vi "camera_imaging_source_MAIN.vi"() -> ()   [LabVIEW 2024]
panel:
  out "Camera Ready":bool
  in  "Live":bool
  in  "Camera Properties":bool
  in  "Stop Camera":bool
  out "Image":T1(plugin-control)
  in  "ICImagingControl":refnum<k7>(container)
  in  "Configuration File Path":path
  in  "Grab Image":bool
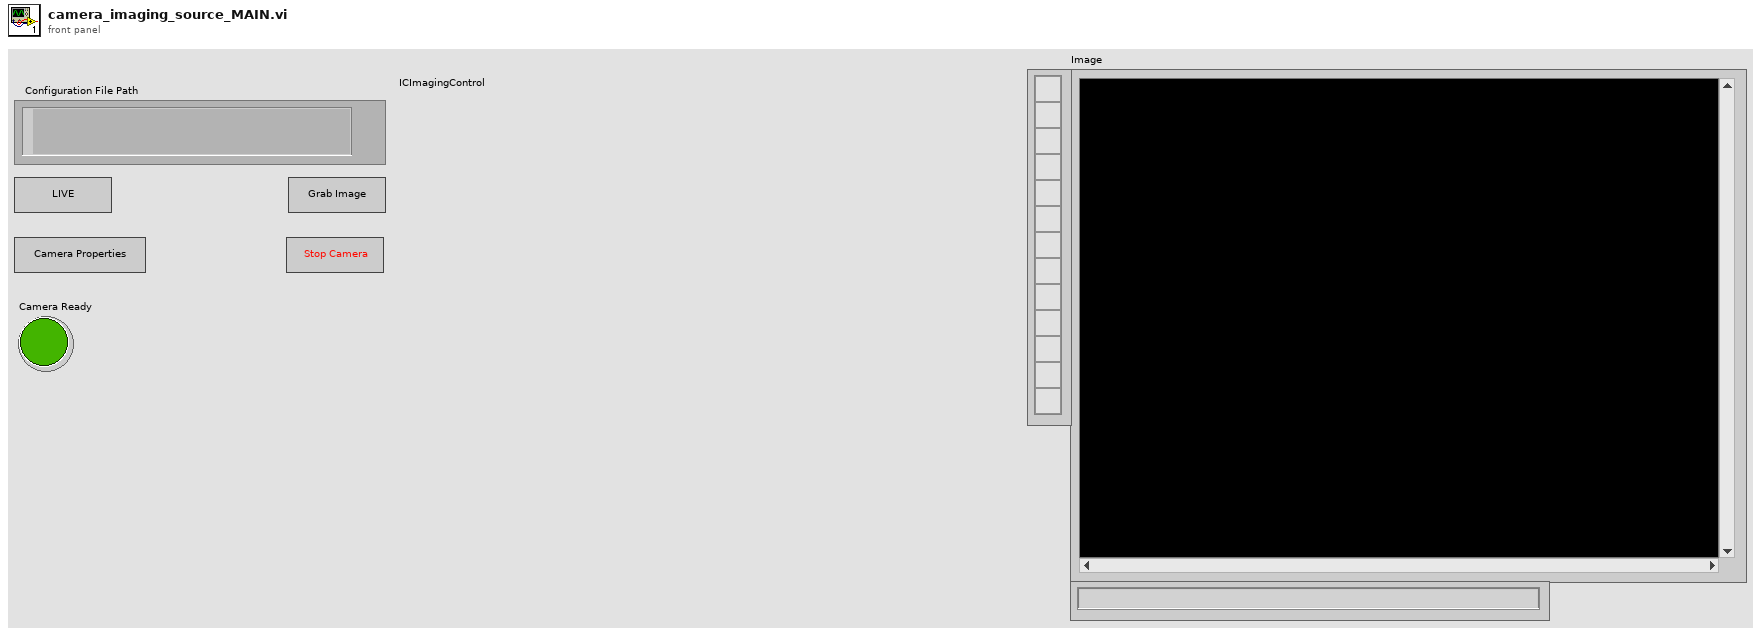
[diagram p1: front panel]
types:
  T1 = typedef "IMAQ Image.ctl" = refnum<image>
  T2 = enum16{"Init", "Idle", "Open Properties", "Grab Image", "Stop All", "Set Live"}
  T3 = enum16{"Init", "Idle", "Open Properties", "Grab Image", "Stop All"}
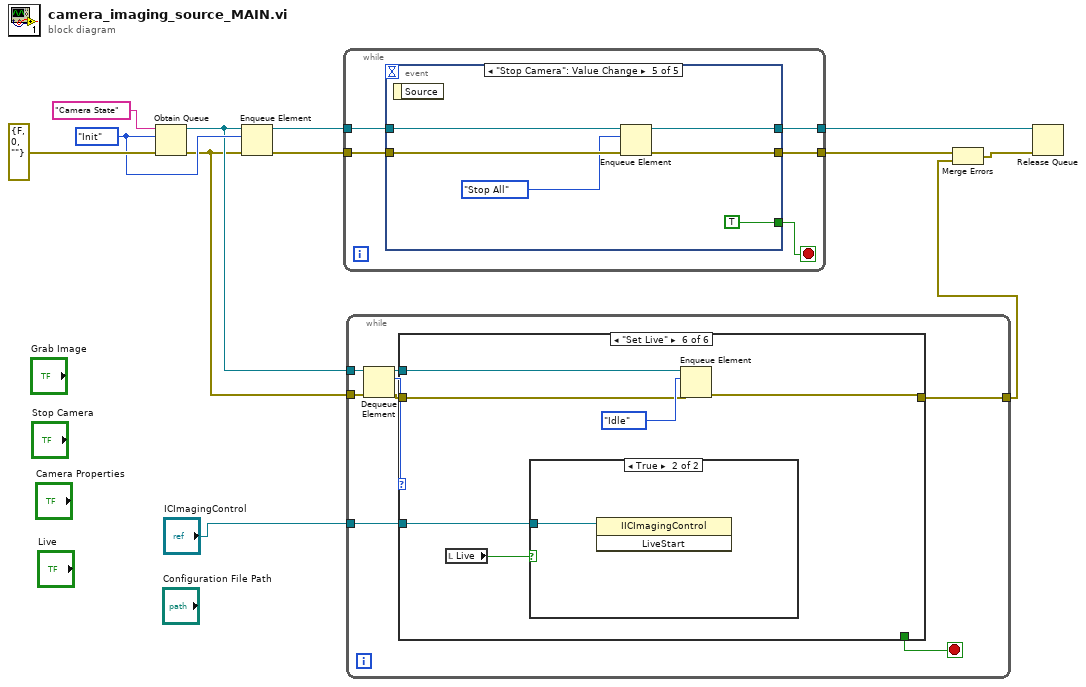
[diagram p0: block diagram]
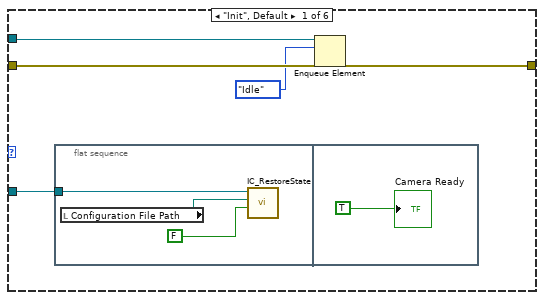
[diagram p2: hidden frame]
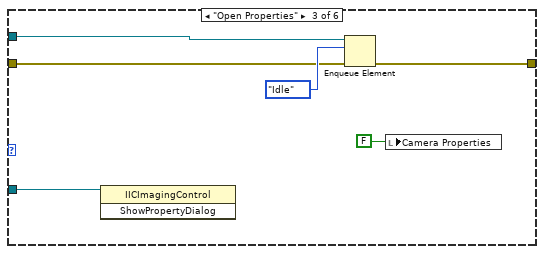
[diagram p4: hidden frame]
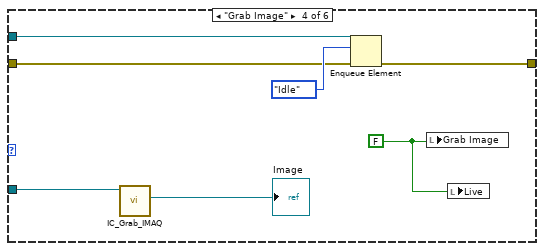
[diagram p5: hidden frame]
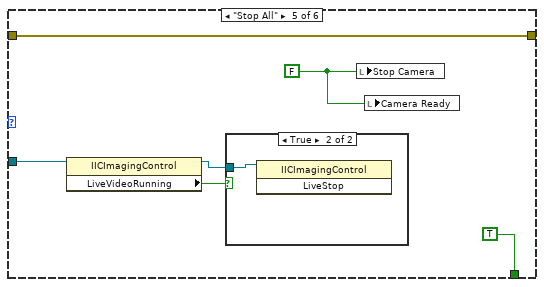
[diagram p6: hidden frame]
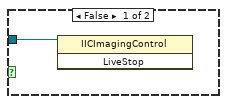
[diagram p8: hidden frame]
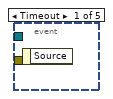
[diagram p9: hidden frame]
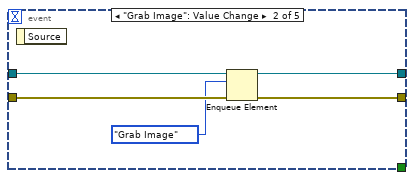
[diagram p10: hidden frame]
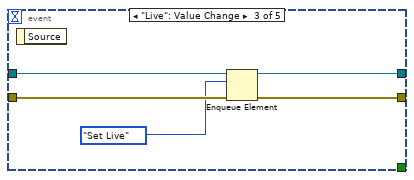
[diagram p11: hidden frame]
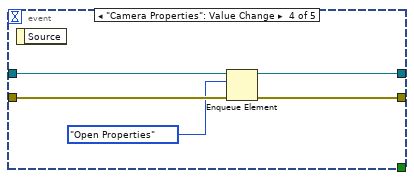
[diagram p12: hidden frame]
diagram:
  w10 = T2."Init"
  n1 = Obtain Queue(name (unnamed)="Camera State", element data type=w10, error in (no error)=errorcluster {"status"=FALSE, "code"=0, "source"=""}) -> (queue out=w9:refnum<queue>, error out=w8:errorcluster)  [unwired: 2 in, 1 out]
  n2 = Enqueue Element(queue=w9, element=w10, error in (no error)=w8) -> (queue out=w6:refnum<queue>, error out=w5:errorcluster)  [unwired: 1 in, 1 out]
  n3 = while {
    tunnel: w6 -> [w17]
    tunnel: w5 -> [w16]
    tunnel: [w15] -> w4
    tunnel: [w14] -> w2
    stop <- w13 stop-if-true
    n4 = event shown="[4] \"Stop Camera\": Value Change" {
      selector: _ -> [_ _ _ _ _]
      dyn-events: _ -> [_ _ _ _ _]
      timeout: _ -> [_ _ _ _ _]
      tunnel: w17 -> [_ w22 w27 w32 w37]
      tunnel: w16 -> [_ w21 w26 w31 w36]
      tunnel: [_ w19 w25 w29 w34] -> w15
      tunnel: [_ w18 w24 w28 w35] -> w14
      tunnel: [_ _ _ _ TRUE] -> w13
      event Timeout {
        n5 = event-data() -> ()  [unwired: 1 in, 1 out]
      }
      event "Grab Image": Value Change {
        n6 = event-data() -> ()  [unwired: 1 in, 1 out]
        n7 = Enqueue Element(queue=w22, element=T3."Grab Image", error in (no error)=w21) -> (queue out=w19:refnum<queue>, error out=w18:errorcluster)  [unwired: 1 in, 1 out]
      }
      event "Live": Value Change {
        n8 = event-data() -> ()  [unwired: 1 in, 1 out]
        n9 = Enqueue Element(queue=w27, element=T2."Set Live", error in (no error)=w26) -> (queue out=w25:refnum<queue>, error out=w24:errorcluster)  [unwired: 1 in, 1 out]
      }
      event "Camera Properties": Value Change {
        n10 = event-data() -> ()  [unwired: 1 in, 1 out]
        n11 = Enqueue Element(queue=w32, element=T3."Open Properties", error in (no error)=w31) -> (queue out=w29:refnum<queue>, error out=w28:errorcluster)  [unwired: 1 in, 1 out]
      }
      event "Stop Camera": Value Change {
        n12 = event-data() -> ()  [unwired: 1 in, 1 out]
        n13 = Enqueue Element(queue=w37, element=T3."Stop All", error in (no error)=w36) -> (queue out=w34:refnum<queue>, error out=w35:errorcluster)  [unwired: 1 in, 1 out]
      }
    }
  }
  n14 = while {
    tunnel: w9 -> [w46]
    tunnel: w8 -> [w45]
    tunnel: "ICImagingControl" -> [w43]
    tunnel: [w42] -> w3
    stop <- w40 stop-if-true
    n15 = Dequeue Element(queue=w46, error in (no error)=w45) -> (queue out=w39:refnum<queue>, element=w44:T2, error out=w41:errorcluster)  [unwired: 1 in, 1 out]
    n16 = case shown="\"Set Live\"" w44 {
      tunnel: w43 -> [w47 _ w62 w69 w74 w82]
      tunnel: [w50 w56 w58 w65 w71 w77] -> w42
      tunnel: w41 -> [w51 w56 w59 w66 w71 w78]
      tunnel: [_ _ _ _ TRUE _] -> w40
      tunnel: w39 -> [w49 _ w60 w64 _ w79]
      frame "Init", Default {
        n17 = flat-sequence {
          tunnel: w47 -> [w52]
          frame #0 {
            n18 = local read "Configuration File Path"() -> (w54:path)
            n19 = call <userlib>:"IC_RestoreState.vi"("Color"=FALSE, "File Path"=w54, "ICImagingControl"=w52) -> ()  [unwired: 1 in, 2 out]
          }
          frame #1 {
            "Camera Ready" <- TRUE
          }
        }
        n20 = Enqueue Element(queue=w49, element=T3."Idle", error in (no error)=w51) -> (error out=w50:errorcluster)  [unwired: 1 in, 2 out]
      }
      frame "Idle" {
      }
      frame "Open Properties" {
        n21 = invoke class="IICImagingControl" method="ShowPropertyDialog"(reference=w62) -> ()  [unwired: 2 in, 3 out]
        n22 = Enqueue Element(queue=w60, element=T3."Idle", error in (no error)=w59) -> (error out=w58:errorcluster)  [unwired: 1 in, 2 out]
        n23 = local write "Camera Properties"(FALSE) -> ()
      }
      frame "Grab Image" {
        w63 = FALSE
        n24 = call <userlib>:"IC_Grab_IMAQ.vi"("ICImagingControl In"=w69) -> ("Image Out"=→"Image":T1)  [unwired: 2 in, 3 out]
        n25 = Enqueue Element(queue=w64, element=T3."Idle", error in (no error)=w66) -> (error out=w65:errorcluster)  [unwired: 1 in, 2 out]
        n26 = local write "Grab Image"(w63) -> ()
        n27 = local write "Live"(w63) -> ()
      }
      frame "Stop All" {
        w70 = FALSE
        n28 = property class="IICImagingControl"(reference=w74) -> (reference out=w72:refnum<k7>, "LiveVideoRunning"=w73:bool)  [unwired: 1 in, 1 out]
        n29 = case shown="True" w73 {
          tunnel: w72 -> [_ w76]
          frame False {
          }
          frame True {
            n30 = invoke class="IICImagingControl" method="LiveStop"(reference=w76) -> ()  [unwired: 2 in, 3 out]
          }
        }
        n31 = local write "Stop Camera"(w70) -> ()
        n32 = local write "Camera Ready"(w70) -> ()
      }
      frame "Set Live" {
        n33 = local read "Live"() -> (w81:bool)
        n34 = case shown="True" w81 {
          tunnel: w82 -> [w83 w84]
          frame False {
            n35 = invoke class="IICImagingControl" method="LiveStop"(reference=w83) -> ()  [unwired: 2 in, 3 out]
          }
          frame True {
            n36 = invoke class="IICImagingControl" method="LiveStart"(reference=w84) -> ()  [unwired: 2 in, 3 out]
          }
        }
        n37 = Enqueue Element(queue=w79, element=T3."Idle", error in (no error)=w78) -> (error out=w77:errorcluster)  [unwired: 1 in, 2 out]
      }
    }
  }
  n38 = Merge Errors(w2, w3) -> (w1:errorcluster)
  n39 = Release Queue(queue=w4, error in (no error)=w1) -> ()  [unwired: 1 in, 3 out]
